vi "Event Handle Loop_Get Ctl Refnum By Label.vi"(8 "error in (no error)":errorcluster, 10 "Label":string, 11 "QTab Class in":refnum<class "QTab Class.lvclass">) -> (0 "error out":errorcluster, 2 "Ctl Refnum":refnum<vi>, 3 "QTab Class out":refnum<class "QTab Class.lvclass">)   [LabVIEW 2020, in "QTab.lvlib" / "QTab Class.lvclass"]
uses:
  QTab Class.lvclass
  QTab Class.lvclass/QTab Class.ctl
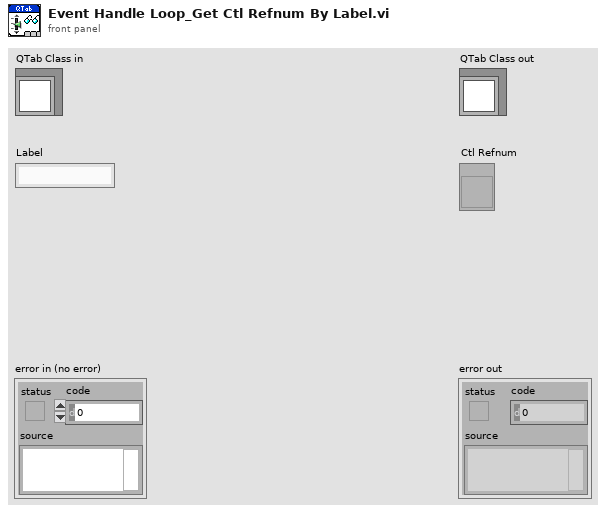
[diagram p1: front panel]
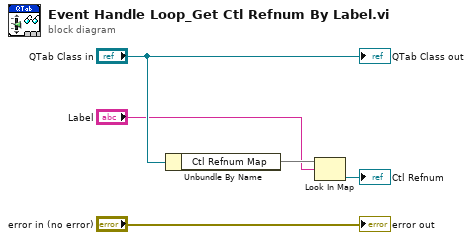
[diagram p0: block diagram]
diagram:
  n1 = Unbundle By Name("QTab Class in") -> ("Ctl Refnum Map"=w4:map{string, refnum<vi>})
  n2 = Look In Map(map=w4, key="Label") -> (value=→"Ctl Refnum":refnum<vi>)  [unwired: 1 in, 1 out]
  "error out" <- "error in (no error)"
  "QTab Class out" <- "QTab Class in"
